vi "Execution Monitor RTM.vi"(8 "error in (no error)":errorcluster, 11 "Node Ptr":u64 format="%.0x") -> (0 "error out":errorcluster)   [LabVIEW 2020, in "AIM MIL-STD-1553 System Explorer.lvlib" / "Implementation.lvlib"]
uses:
  Implementation.lvlib
  Scripting/AIM MIL-STD-1553 Scripting.lvlib
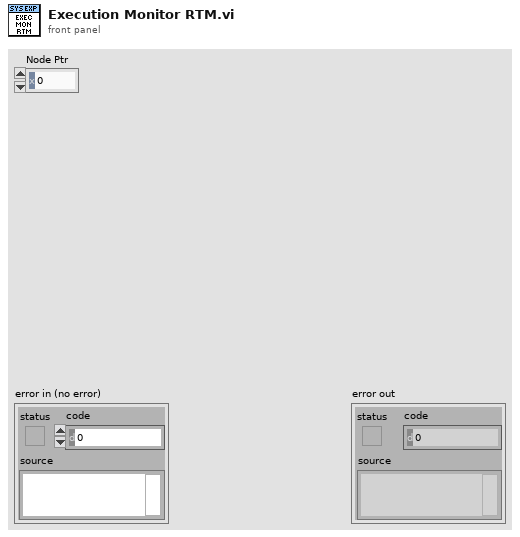
[diagram p1: front panel]
types:
  T1 = typedef "Custom Device API.lvlib/Custom Device Item Ref.ctl" = u64
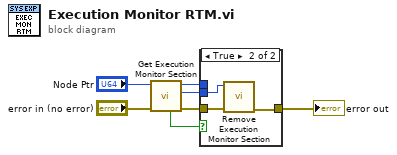
[diagram p0: block diagram]
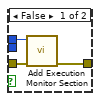
[diagram p2: hidden frame]
diagram:
  n1 = call "Get Execution Monitor Section.vi"("error in"="error in (no error)", "custom device"="Node Ptr") -> ("error out"=w4:errorcluster, "execution monitor section"=w1:T1, "custom device out"=w2:T1, "Found"=w3:bool)  [unwired: 6 in]
  n2 = case shown="True" w3 {
    tunnel: [w10 w12] -> w7
    tunnel: w4 -> [w9 w13]
    tunnel: w2 -> [w8 _]
    tunnel: w1 -> [_ w11]
    frame False {
      n3 = call "Add Execution Monitor Section.vi"("error in"=w9, "custom device"=w8) -> ("error out"=w10:errorcluster)  [unwired: 7 in, 2 out]
    }
    frame True {
      n4 = call "Remove Execution Monitor Section.vi"("error in"=w13, "execution monitor section"=w11) -> ("error out"=w12:errorcluster)  [unwired: 9 in]
    }
  }
  "error out" <- w7
